vi "Log.vi"(1 "Method":enum16{"Init", "Log"}(ring)=enum."Log", 2 "Data":string, 3 "ListBox in":refnum<vi>) -> ()   [LabVIEW 2014]
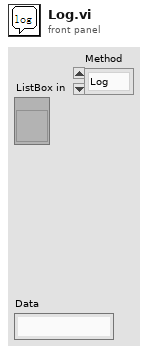
[diagram p1: front panel]
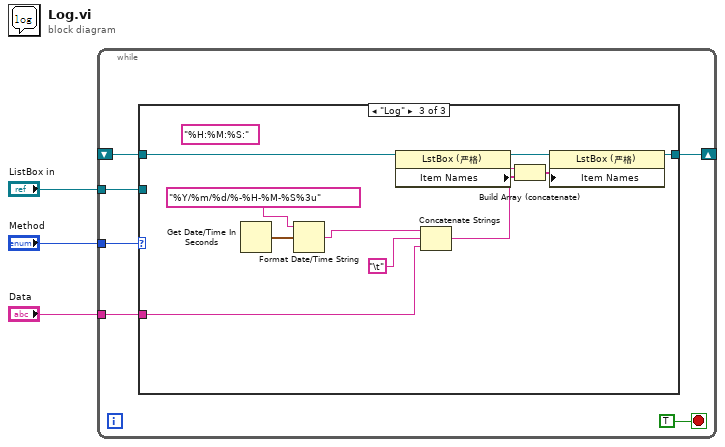
[diagram p0: block diagram]
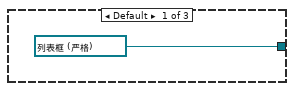
[diagram p2: hidden frame]
diagram:
  n1 = while {
    shift-right: [w6] -> _
    shift-left: _ -> [w8]
    tunnel: "Method" -> [w7]
    tunnel: "ListBox in" -> [w5]
    tunnel: "Data" -> [w4]
    stop <- TRUE stop-if-true
    n2 = case shown="\"Log\"" w7 {
      tunnel: w8 -> [_ _ w17]
      tunnel: [refnum<vi> refnum ("ListBox in") w11 w16] -> w6
      tunnel: w5 -> [_ w11 _]
      tunnel: w4 -> [_ _ w15]
      frame Default {
      }
      frame "Init" {
      }
      frame "Log" {
        (unwired) "%H:%M:%S:" ("time format string (%c)")
        n3 = Get Date/Time In Seconds() -> (seconds since 1Jan1904=w14:timestamp)
        n4 = Format Date/Time String(time format string (%c)="%Y/%m/%d/%-%H-%M-%S%3u" ("时间格式字符串(%c)"), seconds (now)=w14) -> (date/time string=w12:string)  [unwired: 1 in]
        n5 = property on="Property Node" class="LstBox (严格)"(reference=w17) -> (reference out=w22:refnum<vi>, "Item Names"=w19:string[])  [unwired: 1 in, 1 out]
        n6 = Concatenate Strings(w12, "\t", w15) -> (w20:string)
        n7 = Build Array (concatenate)(w20, w19) -> (w21:string[])
        n8 = property on="Property Node" class="LstBox (严格)"(reference=w22, "Item Names"=w21) -> (reference out=w16:refnum<vi>)  [unwired: 1 in, 1 out]
      }
    }
  }
